vi "AssertControlInVisible_Tests.vi"(8 "error in (no error)":errorcluster) -> (0 "error out":errorcluster)   [LabVIEW 2016, in "DronaTest.lvlib"]
uses:
  DronaTest.lvlib
  APIs/Stimulus/ControlValue/ValueSignalByPathString.vi
  APIs/Assert/AssertControlProperty/AssertControlVisible/AssertInvisible.vi
  Drona.lvlib
  APIs/Stimulus/ControlValue/ControlValue.lvlib
  <vilib>/addons/_JKI Toolkits/Caraya/classes/Test/Test.lvclass
  APIs/Assert/AssertControlProperty/AssertControlVisible/AssertControlVisible.lvlib
  <vilib>/addons/_JKI Toolkits/Caraya/classes/Assert/Assert.lvclass
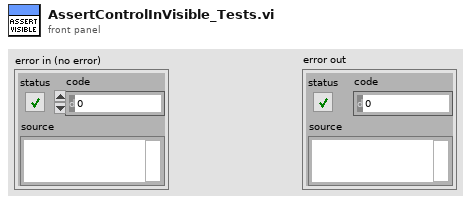
[diagram p1: front panel]
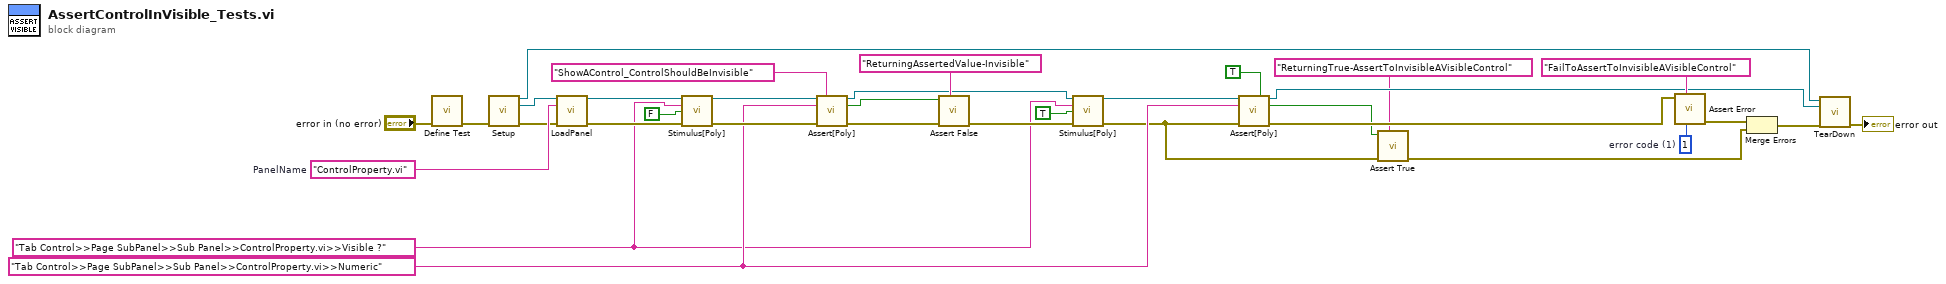
[diagram p0: block diagram]
diagram:
  w11 = 1  # error code (1)
  w13 = "Tab Control>>Page SubPanel>>Sub Panel>>ControlProperty.vi>>Numeric" ("Control Path")
  w6 = "Tab Control>>Page SubPanel>>Sub Panel>>ControlProperty.vi>>Visible ?" ("Control Path")
  w32 = "ControlProperty.vi"  # PanelName
  n1 = call <vilib>:"Define Test.vi"("error in (no error)"="error in (no error)") -> ("error out"=w26:errorcluster)  [unwired: 9 in, 1 out]
  n2 = call "Setup.vi"("error in (no error)"=w26) -> ("Application Ref"=w22:refnum<vi>, "VI out"=w27:refnum<vi>, "error out"=w28:errorcluster)  [unwired: 12 in]
  n3 = call "LoadPanel.vi"("VI in"=w27, "Item Name"=w32, "error in (no error)"=w28) -> ("VI out"=w19:refnum<vi>, "error out"=w29:errorcluster)  [unwired: 11 in]
  n4 = call-poly "Stimulus[Poly].vi"("VI Reference In"=w19, "Control Path"=w6, "Value (Signaling)"=FALSE, "error in"=w29) -> ("VI Reference Out"=w31:refnum<vi>, "error out"=w21:errorcluster)  [unwired: 10 in]
  n5 = call-poly "Assert[Poly].vi"("VI Reference In"=w31, "Label"="ShowAControl_ControlShouldBeInvisible" ("string"), "Control Path"=w13, "Error In"=w21) -> ("VI Reference Out"=w8:refnum<vi>, "Asserted Value"=w20:bool, "Error Out"=w24:errorcluster)  [unwired: 9 in]
  n6 = call <vilib>:"Assert False.vi"("Label"="ReturningAssertedValue-Invisible", "error in (no error)"=w24, "False?"=w20) -> ("error out"=w9:errorcluster)  [unwired: 7 in, 1 out]
  n7 = call-poly "Stimulus[Poly].vi"("VI Reference In"=w8, "Control Path"=w6, "Value (Signaling)"=TRUE, "error in"=w9) -> ("VI Reference Out"=w7:refnum<vi>, "error out"=w5:errorcluster)  [unwired: 10 in]
  n8 = call-poly "Assert[Poly].vi"("VI Reference In"=w7, "Assert Only? (F)"=TRUE, "Control Path"=w13, "Error In"=w5) -> ("VI Reference Out"=w12:refnum<vi>, "Asserted Value"=w3:bool, "Error Out"=w17:errorcluster)  [unwired: 9 in]
  n9 = call <vilib>:"Assert True.vi"("Label"="ReturningTrue-AssertToInvisibleAVisibleControl", "error in (no error)"=w5, "True?"=w3) -> ("error out"=w1:errorcluster)  [unwired: 7 in, 1 out]
  n10 = call <vilib>:"Assert Error.vi"("error code (1)"=w11, "Label"="FailToAssertToInvisibleAVisibleControl", "Error?"=w17) -> ("error out"=w16:errorcluster)  [unwired: 7 in, 1 out]
  n11 = Merge Errors(w16, w1) -> (w2:errorcluster)
  n12 = call "TearDown.vi"("Application Ref"=w22, "VI in"=w12, "error in (no error)"=w2) -> ("error out"=→"error out":errorcluster)  [unwired: 12 in]
